vi "fgv.vi"(7 "Command":T2, 11 "StartArgs":T1) -> (2 "Added":refnum<user-event>, 3 "Modules":T1[](array[typedef]))   [LabVIEW 2024, in "FGVWithEventTrace.lvclass"]
uses:
  FGVWithEventTrace.lvclass
  Command.ctl
  DebugTraceHandle/StartArgs.ctl
  DebugTraceHandle/DebugTraceHandle.lvclass
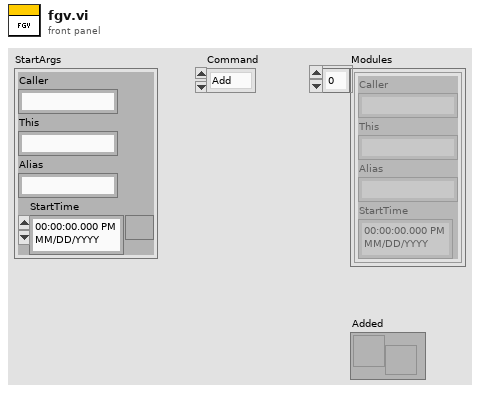
[diagram p1: front panel]
types:
  T1 = typedef "DebugTraceHandle.lvclass/StartArgs.ctl" = cluster{"Caller":string, "This":string, "Alias":string, "StartTime":timestamp}
  T2 = typedef "FGVWithEventTrace.lvclass/Command.ctl" = enum16{"Add", "Get", "Remove", "Clear"}
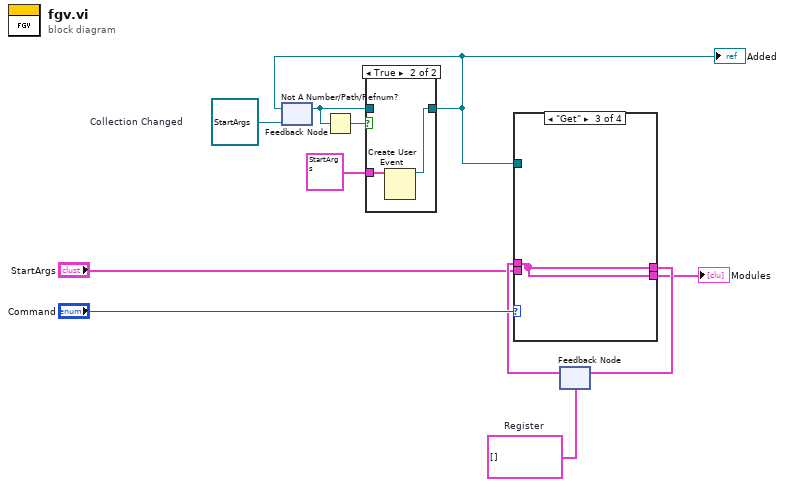
[diagram p0: block diagram]
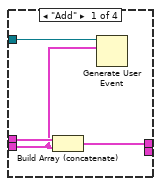
[diagram p3: hidden frame]
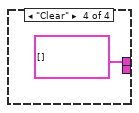
[diagram p5: hidden frame]
diagram:
  w7 = refnum<user-event> refnum  # Collection Changed
  w8 = T1[] []  # Register
  n1 = feedback #1(w7) -> (w5:refnum<user-event>)
  n2 = Not A Number/Path/Refnum?(number/path/refnum=w5) -> (NaN/Path/Refnum?=w6:bool)
  n3 = case shown="True" w6 {
    tunnel: [w12 w14] -> w2
    tunnel: w5 -> [w12 _]
    tunnel: T1 {"Caller"="", "This"="", "Alias"="", "StartTime"=timestamp(0 s since 1904-01-01)} ("StartArgs") -> [_ w13]
    frame False {
    }
    frame True {
      n4 = Create User Event(user event datatype=w13) -> (user event=w14:refnum<user-event>)  [unwired: 1 in, 1 out]
    }
  }
  "Added" <- w2
  n5 = feedback-in #1(w2) -> ()
  n6 = feedback #2(w8) -> (w9:T1[])
  n7 = case shown="\"Get\"" "Command" {
    tunnel: [w16 w19 w20 T1[] []] -> w10
    tunnel: w9 -> [w18 w19 w20 _]
    tunnel: "StartArgs" -> [w15 _ _ _]
    tunnel: [_ _ w20 _] -> w1
    tunnel: w2 -> [w17 _ _ _]
    frame "Add" {
      n8 = Build Array (concatenate)(w18, w15) -> (w16:T1[])
      n9 = Generate User Event(user event=w17, event data cluster=w15) -> ()  [unwired: 2 in, 2 out]
    }
    frame "Remove" {
    }
    frame "Get" {
    }
    frame "Clear" {
    }
  }
  "Modules" <- w1
  n10 = feedback-in #2(w10) -> ()
